vi "Add Verbose Explanation.vi"(5 "append":bool, 7 "overwrite":bool, 8 "error in (no error)":errorcluster, 10 "Verbose Explanation":string, 11 "Leaf in":refnum<class "Leaf.lvclass">) -> (0 "error out":errorcluster, 3 "Leaf out":refnum<class "Leaf.lvclass">)   [LabVIEW 2021, in "Bananas.lvlib" / "Leaf.lvclass"]
uses:
  Leaf.lvclass
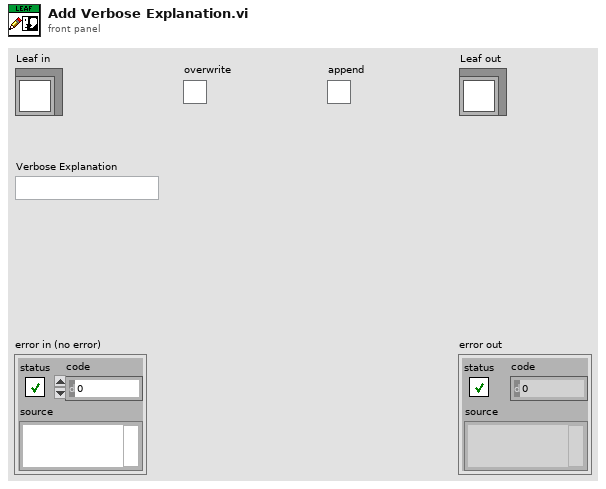
[diagram p1: front panel]
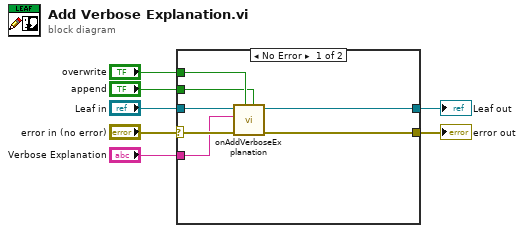
[diagram p0: block diagram]
diagram:
  n1 = case shown="No Error" "error in (no error)" {
    selector: "error in (no error)" -> [w13 w16]
    tunnel: [w8 w16] -> w6
    tunnel: [w9 w15] -> w4
    tunnel: "Leaf in" -> [w14 w15]
    tunnel: "Verbose Explanation" -> [w12 _]
    tunnel: "overwrite" -> [w11 _]
    tunnel: "append" -> [w10 _]
    frame No Error {
      n2 = call-dynamic "onAddVerboseExplanation.vi"("append"=w10, "overwrite"=w11, "error in (no error)"=w13, "Verbose Explanation"=w12, "Leaf in"=w14) -> ("error out"=w8:errorcluster, "Leaf out"=w9:refnum<class "Leaf.lvclass">)  [unwired: 5 in]
    }
    frame Error {
    }
  }
  "error out" <- w6
  "Leaf out" <- w4
